vi "Syringe On.vi"(8 "error in":errorcluster, 11 "SyringeTool":refnum<class "SyringeTool Class.lvclass">) -> (0 "error out":errorcluster, 3 "SyringeTool out":refnum<class "SyringeTool Class.lvclass">)   [LabVIEW 2011, in "SyringeTool Class.lvclass"]
uses:
  SyringeTool Class.lvclass
  WorkTable Class/WorkTable Class.lvclass
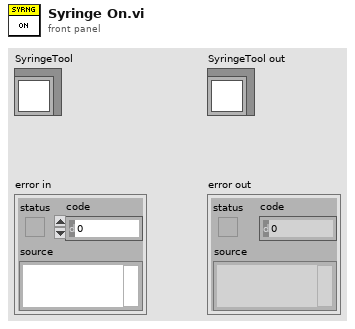
[diagram p1: front panel]
types:
  T1 = typedef "Worktable_Dispenser.ctl" = cluster{"Hardware Path":string, "Enabled":bool}
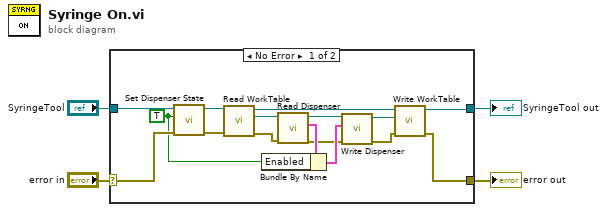
[diagram p0: block diagram]
diagram:
  n1 = case shown="No Error" "error in" {
    selector: "error in" -> [w17 w22]
    tunnel: [w5 w22] -> w3
    tunnel: [w6 w21] -> w1
    tunnel: "SyringeTool" -> [w18 w21]
    frame No Error {
      w13 = TRUE ("On/Off")
      n2 = call-dynamic "Set Dispenser State.vi"("error in (no error)"=w17, "On/Off"=w13, "Gantry Class in"=w18) -> ("error out"=w15:errorcluster, "Gantry Class out"=w16:refnum<class "SyringeTool Class.lvclass">)  [unwired: 7 in]
      n3 = call-dynamic "Read WorkTable.vi"("error in"=w15, "Gantry Class in"=w16) -> ("error out"=w19:errorcluster, "WorkTable Class.lvclass"=w20:refnum<class "WorkTable Class.lvclass">, "Gantry Class out"=w7:refnum<class "SyringeTool Class.lvclass">)  [unwired: 7 in]
      n4 = call-dynamic "Read Dispenser.vi"("error in (no error)"=w19, "WorkTable Class in"=w20) -> ("error out"=w10:errorcluster, "Dispenser"=w14:T1, "WorkTable Class out"=w11:refnum<class "WorkTable Class.lvclass">)  [unwired: 7 in]
      n5 = Bundle By Name(cluster=w14, "Enabled"=w13) -> (w12:T1)
      n6 = call-dynamic "Write Dispenser.vi"("error in (no error)"=w10, "Dispenser"=w12, "WorkTable Class in"=w11) -> ("error out"=w9:errorcluster, "WorkTable Class out"=w8:refnum<class "WorkTable Class.lvclass">)  [unwired: 7 in]
      n7 = call-dynamic "Write WorkTable.vi"("error in (no error)"=w9, "WorkTable Class.lvclass"=w8, "Gantry Class in"=w7) -> ("error out"=w5:errorcluster, "Gantry Class out"=w6:refnum<class "SyringeTool Class.lvclass">)  [unwired: 7 in]
    }
    frame Error {
    }
  }
  "error out" <- w3
  "SyringeTool out" <- w1
